vi "save pre-launch status.vi"(6 "save pre-launch status":bool, 7 "vi ref":refnum<vi>, 8 "error in (no error)":errorcluster, 11 "status control id":i32) -> (0 "error out":errorcluster)   [LabVIEW 2024, in "status manager.lvlib"]
uses:
  status manager.lvlib
  <vilib>/Utility/error.llb/Trim Whitespace One-Sided.vi
  <vilib>/Hampel Software Engineering/HSE Logger/hse-logger.lvlib
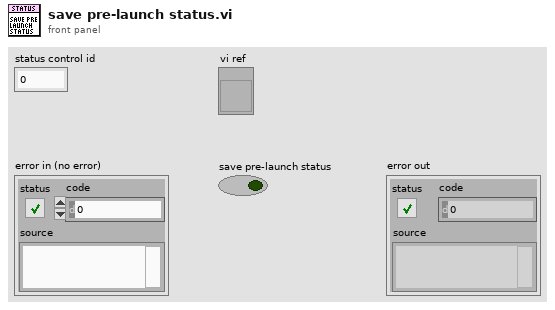
[diagram p1: front panel]
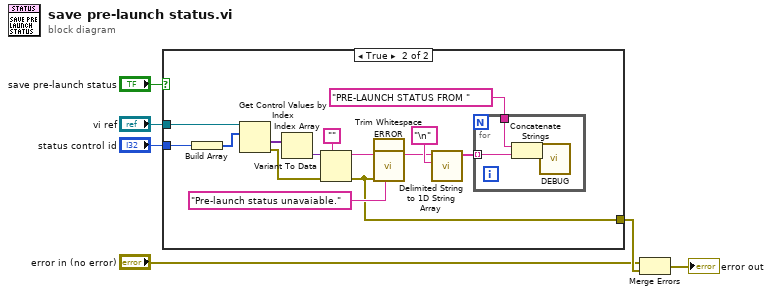
[diagram p0: block diagram]
diagram:
  n1 = case shown="True" "save pre-launch status" {
    tunnel: "vi ref" -> [_ w20]
    tunnel: "status control id" -> [_ w9]
    tunnel: [_ w7] -> w3
    frame False {
    }
    frame True {
      n2 = Build Array(w9) -> (w10:i32[])
      n3 = Get Control Values by Index(0:w20, 1:w10) -> (10:w11:variant[], 11:w14:errorcluster)  [unwired: 1 in]
      n4 = Index Array(array=w11) -> (element=w12:variant)  [unwired: 1 in]
      n5 = Variant To Data(error in=w14, type="", Variant=w12) -> (data=w16:string, error out=w7:errorcluster)
      n6 = call <vilib>:"Trim Whitespace.vi"("string"=w16) -> ("trimmed string"=w8:string)  [unwired: 1 in]
      n7 = call <vilib>:"ERROR.vi"("Message"="Pre-launch status unavaiable.", "error in"=w7) -> ()  [unwired: 9 in, 1 out]
      n8 = call <vilib>:"Delimited String to 1D String Array.vi"("delimiter"="\n", "delimited string"=w8) -> ("string array"=w18:string[])  [unwired: 9 in]
      n9 = for {
        tunnel: w18 -> [w22] mode=indexing
        tunnel: "PRE-LAUNCH STATUS FROM " -> [w23]
        n10 = Concatenate Strings(w23, w22) -> (w21:string)
        n11 = call <vilib>:"DEBUG.vi"("Message"=w21) -> ()  [unwired: 10 in, 1 out]
      }
    }
  }
  n12 = Merge Errors("error in (no error)", w3) -> (→"error out":errorcluster)
